vi "scale CAD in xy graph.vi"(1 "XY Graph":refnum<vi>, 5 "xy graph data":cluster{"X Out":sgl[], "Y Out":sgl[]}[](array[cluster]), 11 "error in (no error)":errorcluster) -> (15 "error out":errorcluster)   [LabVIEW 2013, in "Manipulate IPF.lvlib"]
uses:
  Manipulate IPF.lvlib
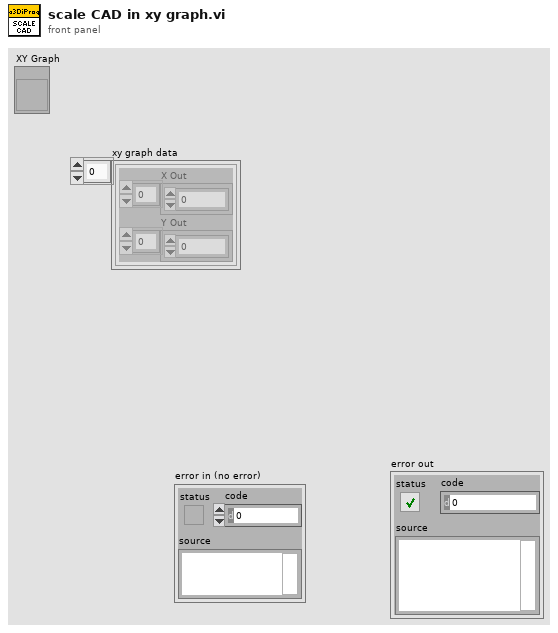
[diagram p1: front panel]
types:
  T1 = typedef "LVPoint32TypeDef.ctl" = cluster{"Horizontal":i32, "Vertical":i32}
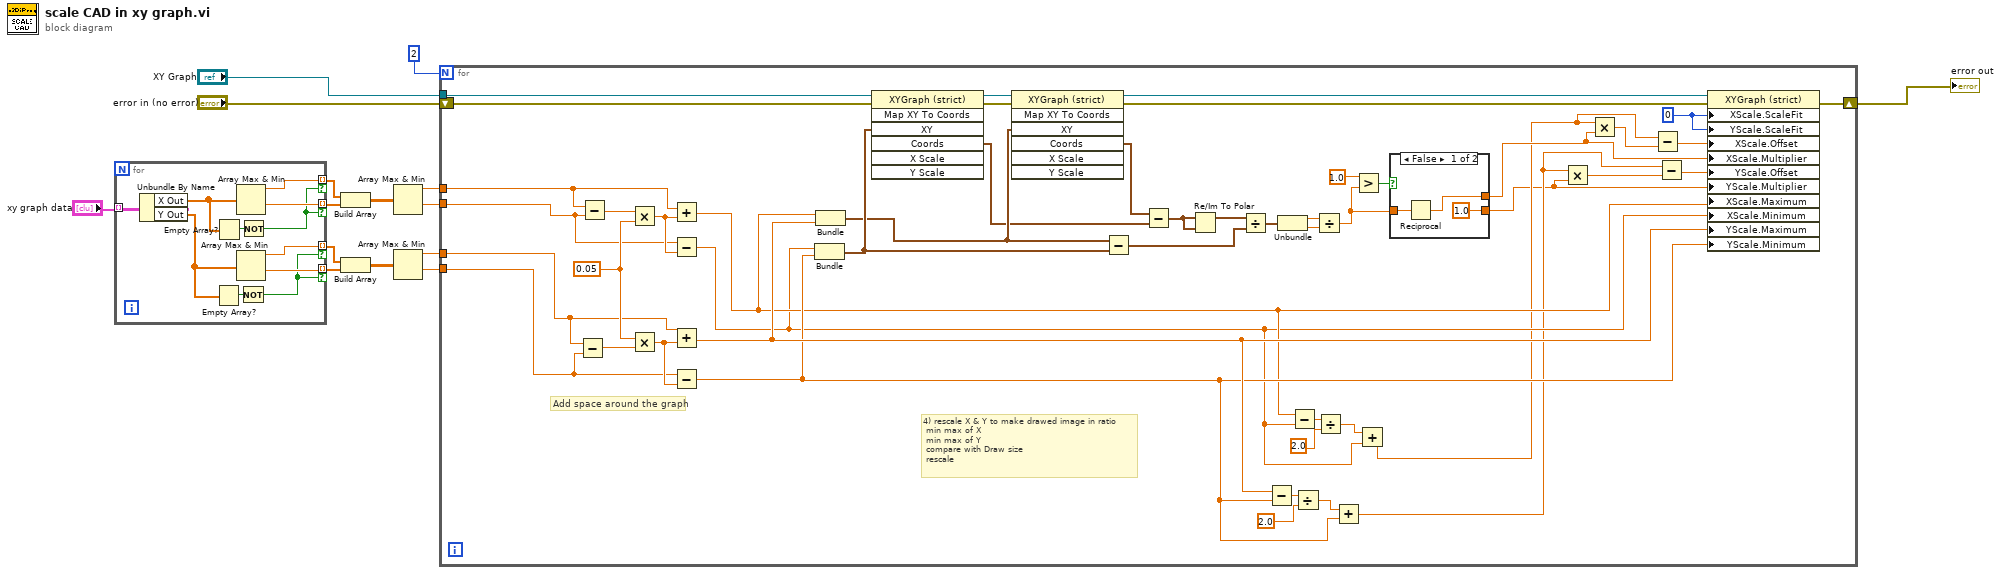
[diagram p0: block diagram]
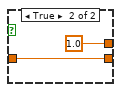
[diagram p2: hidden frame]
diagram:
  n1 = for {
    tunnel: [w26] -> w12 mode=indexing if=w19
    tunnel: [w25] -> w11 mode=indexing if=w19
    tunnel: [w24] -> w8 mode=indexing if=w16
    tunnel: [w23] -> w7 mode=indexing if=w16
    tunnel: "xy graph data" -> [w22] mode=indexing
    n2 = Unbundle By Name(w22) -> ("X Out"=w20:sgl[], "Y Out"=w17:sgl[])
    n3 = Empty Array?(array=w17) -> (empty?=w18:bool)
    n4 = Empty Array?(array=w20) -> (empty?=w21:bool)
    n5 = Array Max & Min(array=w20) -> (max value=w26:sgl, min value=w25:sgl)  [unwired: 2 out]
    n6 = Array Max & Min(array=w17) -> (max value=w24:sgl, min value=w23:sgl)  [unwired: 2 out]
    n7 = Not(x=w18) -> (.not. x?=w16:bool)
    n8 = Not(x=w21) -> (.not. x?=w19:bool)
  }
  n9 = Build Array(w12, w11) -> (w10:sgl[][])
  n10 = Build Array(w8, w7) -> (w9:sgl[][])
  n11 = Array Max & Min(array=w10) -> (max value=w2:sgl, min value=w3:sgl)  [unwired: 2 out]
  n12 = Array Max & Min(array=w9) -> (max value=w4:sgl, min value=w5:sgl)  [unwired: 2 out]
  n13 = for {
    N: 2 -> [_]
    tunnel: w2 -> [w49]
    tunnel: w3 -> [w48]
    tunnel: w5 -> [w47]
    tunnel: w4 -> [w46]
    shift-right: [w45] -> w14
    shift-left: "error in (no error)" -> [w68]
    tunnel: "XY Graph" -> [w44]
    w72 = 0.05
    w69 = 0
    # "Add space around the graph"
    # "4) rescale X & Y to make drawed image in ratio\n min max of X\n min max of Y\n compare with Draw size\n rescale"
    n14 = Subtract(x=w46, y=w47) -> (x-y=w70:sgl)
    n15 = Subtract(x=w49, y=w48) -> (x-y=w71:sgl)
    n16 = Multiply(x=w71, y=w72) -> (x*y=w73:dbl)
    n17 = Multiply(x=w72, y=w70) -> (x*y=w74:dbl)
    n18 = Add(x=w49, y=w73) -> (x+y=w33:dbl)
    n19 = Subtract(x=w48, y=w73) -> (x-y=w31:dbl)
    n20 = Add(x=w46, y=w74) -> (x+y=w37:dbl)
    n21 = Subtract(x=w47, y=w74) -> (x-y=w36:dbl)
    n22 = Bundle(w31, w36) -> (w58:cluster{dbl, dbl})  [unwired: 1 in]
    n23 = Bundle(w33, w37) -> (w57:cluster{dbl, dbl})  [unwired: 1 in]
    n24 = invoke on="Invoke Node" class="XYGraph (strict)" method="Map XY To Coords"(reference=w44, error in=w68, "XY"=w58) -> (reference out=w43:refnum<vi>, error out=w67:errorcluster, "Coords"=w56:T1)  [unwired: 4 in, 4 out]
    n25 = invoke on="Invoke Node" class="XYGraph (strict)" method="Map XY To Coords"(reference=w43, error in=w67, "XY"=w57) -> (reference out=w42:refnum<vi>, error out=w66:errorcluster, "Coords"=w55:T1)  [unwired: 4 in, 4 out]
    n26 = Subtract(x=w57, y=w58) -> (x-y=w59:cluster{dbl, dbl})
    n27 = Subtract(x=w55, y=w56) -> (x-y=w63:T1)
    n28 = Re/Im To Polar(2:w63, 3:w63) -> (1:w64:cluster{"Horizontal":dbl, "Vertical":dbl})  [unwired: 1 out]
    n29 = Divide(x=w64, y=w59) -> (x/y=w60:cluster{dbl, dbl})
    n30 = Subtract(x=w37, y=w36) -> (x-y=w39:dbl)
    n31 = Unbundle(w60) -> (w61:dbl, w62:dbl)
    n32 = Subtract(x=w33, y=w31) -> (x-y=w34:dbl)
    n33 = Divide(x=w39, y=2.0) -> (x/y=w38:dbl)
    n34 = Divide(x=w61, y=w62) -> (x/y=w54:dbl)
    n35 = Divide(x=w34, y=2.0) -> (x/y=w35:dbl)
    n36 = Add(x=w38, y=w36) -> (x+y=w29:dbl)
    n37 = Greater?(x=1.0, y=w54) -> (0:w41:bool)
    n38 = Add(x=w35, y=w31) -> (x+y=w28:dbl)
    n39 = case shown="False" w41 {
      tunnel: w54 -> [w76 w78]
      tunnel: [1.0 w78] -> w27
      tunnel: [w75 1.0] -> w30
      frame False {
        n40 = Reciprocal(x=w76) -> (1/x=w75:dbl)
      }
      frame True {
      }
    }
    n41 = Multiply(x=w29, y=w27) -> (x*y=w53:dbl)
    n42 = Multiply(x=w28, y=w30) -> (x*y=w52:dbl)
    n43 = Subtract(x=w28, y=w52) -> (x-y=w51:dbl)
    n44 = Subtract(x=w29, y=w53) -> (x-y=w50:dbl)
    n45 = property on="Property Node" class="XYGraph (strict)"(reference=w42, error in=w66, "XScale.ScaleFit"=w69, "YScale.ScaleFit"=w69, "XScale.Offset"=w51, "XScale.Multiplier"=w30, "YScale.Offset"=w50, "YScale.Multiplier"=w27, "XScale.Maximum"=w33, "XScale.Minimum"=w31, "YScale.Maximum"=w37, "YScale.Minimum"=w36) -> (error out=w45:errorcluster)  [unwired: 1 out]
  }
  "error out" <- w14
